vi "Move (GOTO) -- subVI.vi"(8 "error in (no error)":errorcluster, 10 "Position":dbl, 11 "VISA Refnum in":refnum<visa-resource-name>) -> (0 "error out":errorcluster)   [LabVIEW 2020, in "Monochromator.lvlib"]
uses:
  Monochromator.lvlib
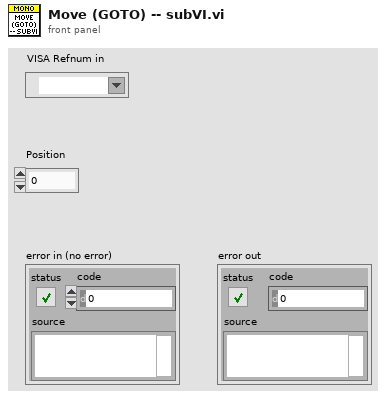
[diagram p1: front panel]
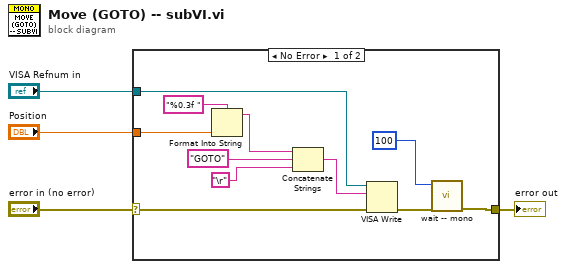
[diagram p0: block diagram]
diagram:
  n1 = case shown="No Error" "error in (no error)" {
    selector: "error in (no error)" -> [w8 w16]
    tunnel: [w5 w16] -> w4
    tunnel: "Position" -> [w13 _]
    tunnel: "VISA Refnum in" -> [w9 _]
    frame No Error {
      n2 = Format Into String(format string="%0.3f ", w13) -> (resulting string=w15:string)  [unwired: 2 in, 1 out]
      n3 = Concatenate Strings(w15, "GOTO" ("string"), "\r") -> (w10:string)
      n4 = VISA Write(VISA resource name=w9, write buffer=w10, error in (no error)=w8) -> (error out=w7:errorcluster)  [unwired: 2 out]
      n5 = call "wait -- mono.vi"("error in (no error)"=w7, "milliseconds to wait"=u32 100) -> ("error out"=w5:errorcluster)  [unwired: 9 in]
    }
    frame Error {
    }
  }
  "error out" <- w4
